vi "BPM-Chassis02 FPGA.vi"() -> ()   [LabVIEW 2011]
uses:
  <vilib>/rvi/eio/common/nirviEmuTemplateMethod_errors.vi
  <vilib>/rvi/Memory/Memory_Emulation/niFpgaMemoryEmulationValidateCache.vi
  <vilib>/rvi/DataTransferAndStorage/Container/Common/niFpgaContainerGetUniqueNameForEmu.vi
  <vilib>/rvi/Memory/Memory_Emulation/nirvimemoryEmulationManagerCache_InsertValue.vi
  <vilib>/Utility/error.llb/Clear Errors.vi
  <vilib>/rvi/Memory/Memory_Emulation/nirvimemoryEmulationManagerCache_GetValue.vi
  <vilib>/rvi/Memory/Memory_Emulation/nirvimemoryEmulationManagerCache_SetValue.vi
  <vilib>/eio/EIONode/EIONode.xnode
  <vilib>/eio/EIOMethodNode/EIOMethodNode.xnode
  <vilib>/rvi/DataTransferAndStorage/Container/XNode/niFpgaContainer.xnode
  <vilib>/rvi/Memory/Memory_Emulation/nirvimemoryEmulation.vi
panel:
  out "period":u32
  out "delay":u32
  out "dperiod":u32
  out "Timestamp":u32 caption="Tick Count(Ticks)"
  out "Mod3/AI3":fxp<+/-,20,5> format="%.17g"
  out "Mod3/AI2":fxp<+/-,20,5> format="%.17g"
  out "Mod1/AI1":fxp<+/-,20,5> format="%.17g"
  out "Mod2/AI3":fxp<+/-,20,5> format="%.17g"
  out "Mod2/AI2":fxp<+/-,20,5> format="%.17g"
  out "Mod2/AI1":fxp<+/-,20,5> format="%.17g"
  out "Mod2/AI0":fxp<+/-,20,5> format="%.17g"
  out "Mod1/AI3":fxp<+/-,20,5> format="%.17g"
  out "Mod1/AI2":fxp<+/-,20,5> format="%.17g"
  out "Mod1/AI0":fxp<+/-,20,5> format="%.17g"
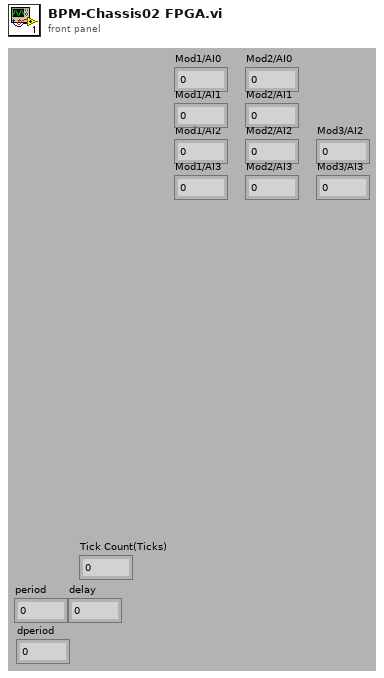
[diagram p1: front panel]
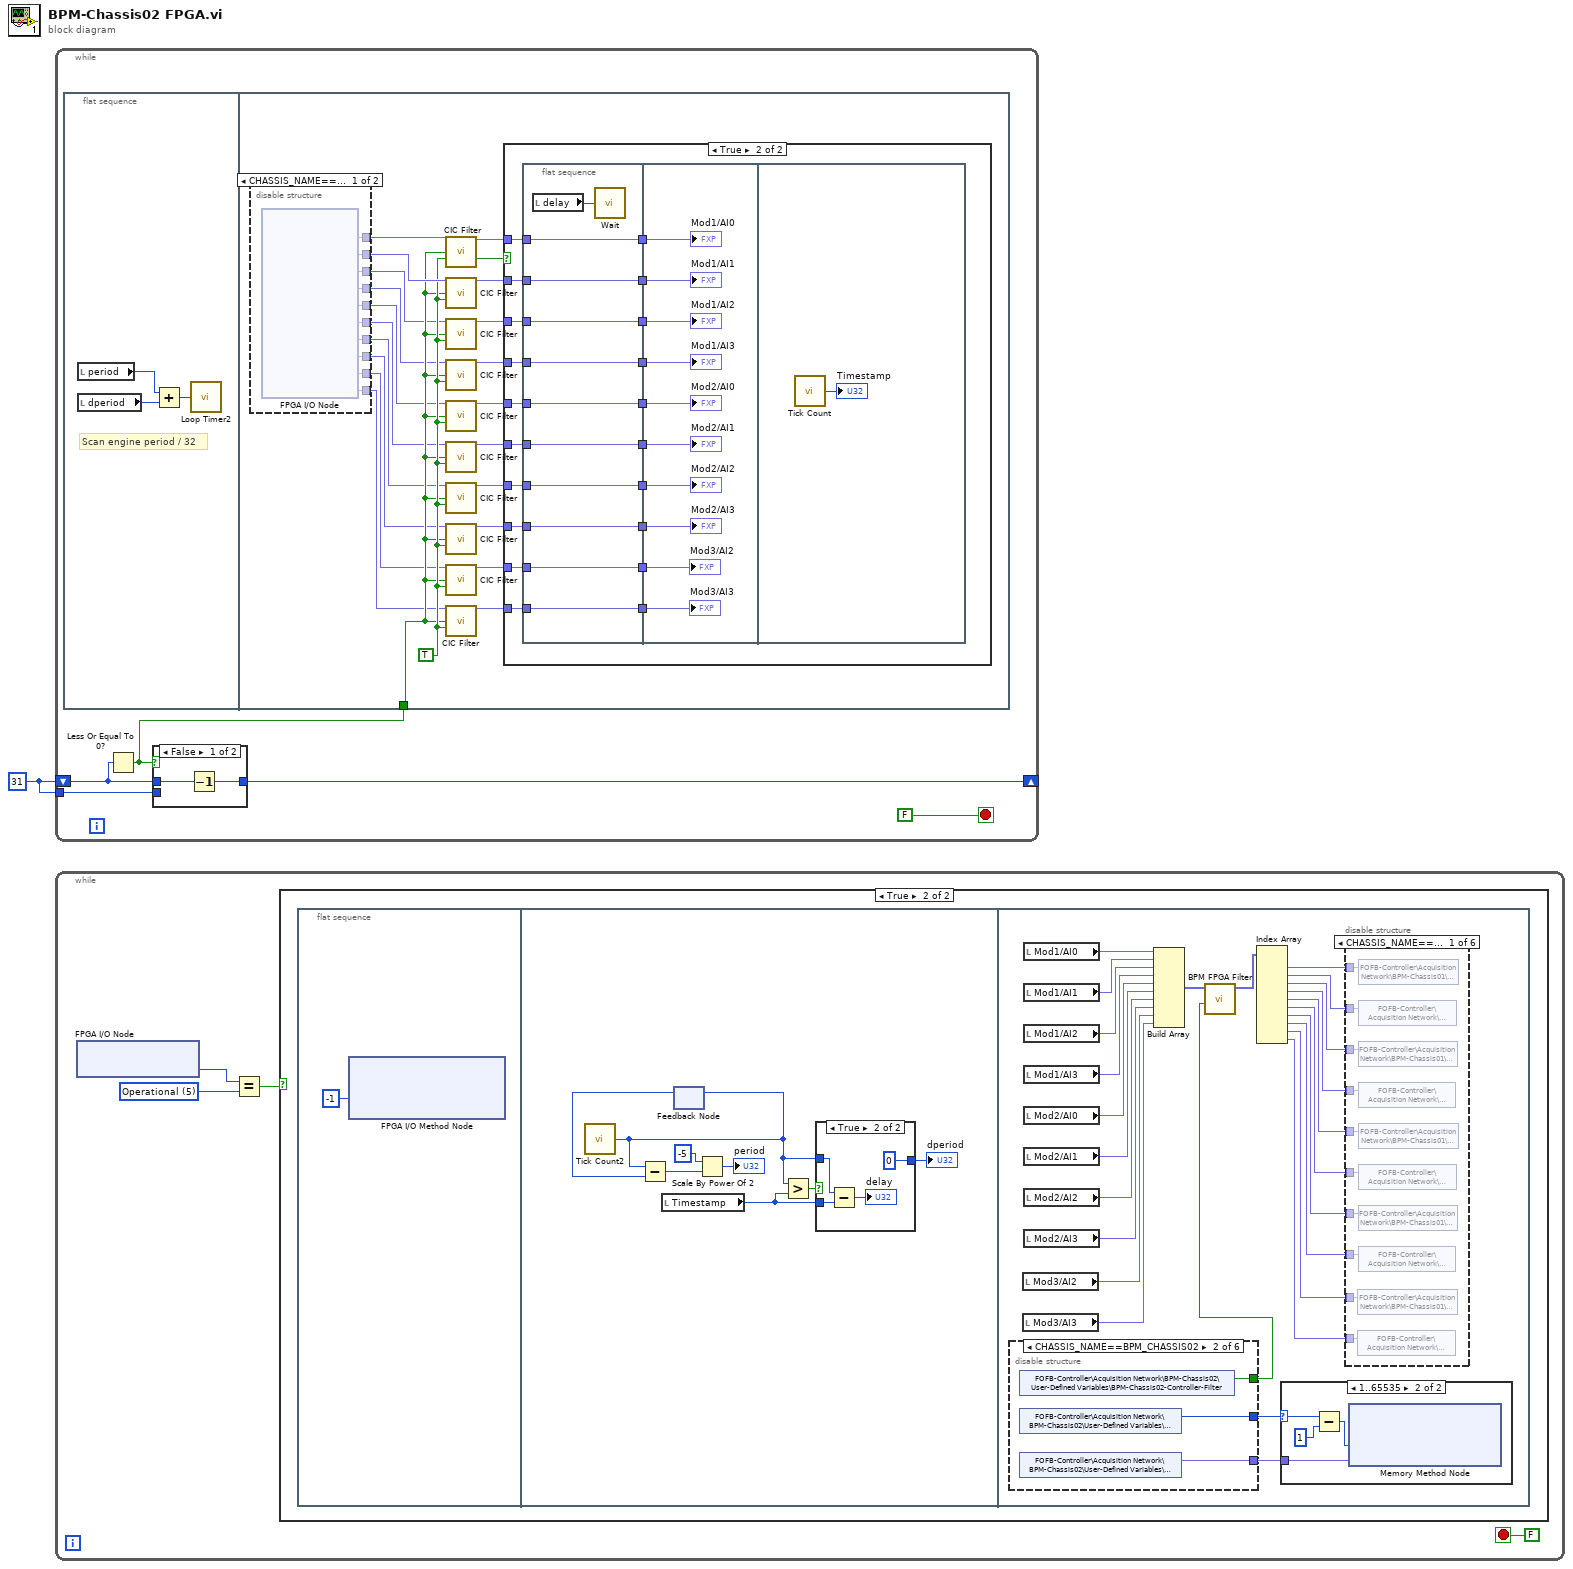
[diagram p0: block diagram]
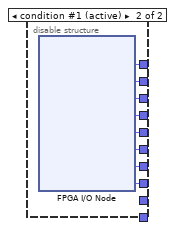
[diagram p3: hidden frame]
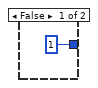
[diagram p6: hidden frame]
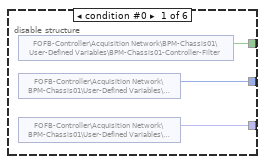
[diagram p8: hidden frame]
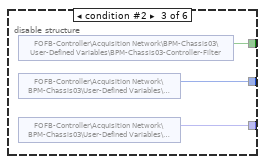
[diagram p9: hidden frame]
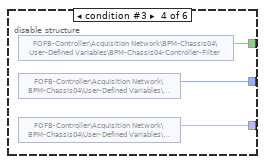
[diagram p10: hidden frame]
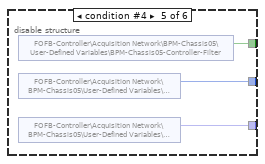
[diagram p11: hidden frame]
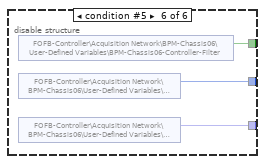
[diagram p12: hidden frame]
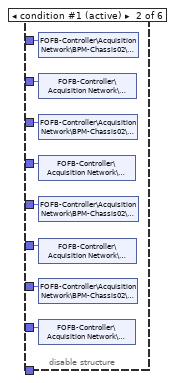
[diagram p13: hidden frame]
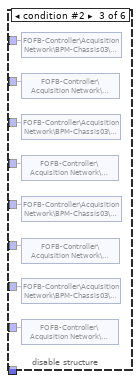
[diagram p14: hidden frame]
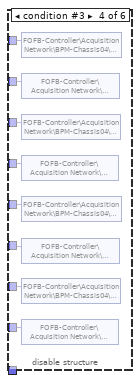
[diagram p15: hidden frame]
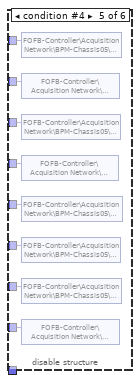
[diagram p16: hidden frame]
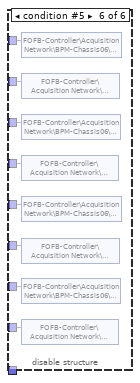
[diagram p17: hidden frame]
diagram:
  w1 = 31
  n1 = while {
    shift-right: [w5] -> _
    shift-left: w1 -> [w4]
    tunnel: w1 -> [w2]
    stop <- FALSE stop-if-true
    n2 = flat-sequence {
      tunnel: w3 -> [w30]
      frame #0 {
        # "Scan engine period / 32"
        n3 = local read "period"() -> (w12:u32)
        n4 = local read "dperiod"() -> (w11:u32)
        n5 = Add(x=w12, y=w11) -> (x+y=w10:u32)
        n6 = call "Loop Timer2"("Count(Ticks)"=w10) -> ()  [unwired: 1 out]
      }
      frame #1 {
        w31 = TRUE ("input valid")
        n7 = disable-structure shown="CHASSIS_NAME==BPM_CHASSIS01" {
          disable-tunnel: [w45 w53] -> w33
          disable-tunnel: [w44 w52] -> w32
          disable-tunnel: [w43 w51] -> w20
          disable-tunnel: [w42 w50] -> w19
          disable-tunnel: [w41 w49] -> w18
          disable-tunnel: [w40 w48] -> w17
          disable-tunnel: [w39 w47] -> w16
          disable-tunnel: [w38 w46] -> w15
          disable-tunnel: [w37 _] -> w14
          disable-tunnel: [w36 _] -> w13
          frame condition #0 {
            n8 = xnode "FPGA I/O Node"() -> ("Mod1/AI0"=w45:fxp<+/-,20,5>, "Mod1/AI1"=w44:fxp<+/-,20,5>, "Mod1/AI2"=w43:fxp<+/-,20,5>, "Mod1/AI3"=w42:fxp<+/-,20,5>, "Mod2/AI0"=w41:fxp<+/-,20,5>, "Mod2/AI1"=w40:fxp<+/-,20,5>, "Mod2/AI2"=w39:fxp<+/-,20,5>, "Mod2/AI3"=w38:fxp<+/-,20,5>, "Mod3/AI2"=w37, "Mod3/AI3"=w36)  [unwired: 10 in, 10 out]
          }
          frame condition #1 (active) {
            n9 = xnode "FPGA I/O Node"() -> ("Mod1/AI0"=w53:fxp<+/-,20,5>, "Mod1/AI1"=w52:fxp<+/-,20,5>, "Mod1/AI2"=w51:fxp<+/-,20,5>, "Mod1/AI3"=w50:fxp<+/-,20,5>, "Mod2/AI0"=w49:fxp<+/-,20,5>, "Mod2/AI1"=w48:fxp<+/-,20,5>, "Mod2/AI2"=w47:fxp<+/-,20,5>, "Mod2/AI3"=w46:fxp<+/-,20,5>)  [unwired: 8 in, 8 out]
          }
        }
        n10 = call "CIC Filter.vi"("input data"=w33, "sample"=w30, "input valid"=w31) -> ("output data"=w34:fxp<+/-,20,5>, "output valid"=w35:bool)  [unwired: 10 in, 1 out]
        n11 = call "CIC Filter.vi"("input data"=w32, "sample"=w30, "input valid"=w31) -> ("output data"=w29:fxp<+/-,20,5>)  [unwired: 10 in, 2 out]
        n12 = call "CIC Filter.vi"("input data"=w20, "sample"=w30, "input valid"=w31) -> ("output data"=w28:fxp<+/-,20,5>)  [unwired: 10 in, 2 out]
        n13 = call "CIC Filter.vi"("input data"=w19, "sample"=w30, "input valid"=w31) -> ("output data"=w27:fxp<+/-,20,5>)  [unwired: 10 in, 2 out]
        n14 = call "CIC Filter.vi"("input data"=w18, "sample"=w30, "input valid"=w31) -> ("output data"=w26:fxp<+/-,20,5>)  [unwired: 10 in, 2 out]
        n15 = call "CIC Filter.vi"("input data"=w17, "sample"=w30, "input valid"=w31) -> ("output data"=w25:fxp<+/-,20,5>)  [unwired: 10 in, 2 out]
        n16 = call "CIC Filter.vi"("input data"=w16, "sample"=w30, "input valid"=w31) -> ("output data"=w24:fxp<+/-,20,5>)  [unwired: 10 in, 2 out]
        n17 = call "CIC Filter.vi"("input data"=w15, "sample"=w30, "input valid"=w31) -> ("output data"=w23:fxp<+/-,20,5>)  [unwired: 10 in, 2 out]
        n18 = call "CIC Filter.vi"("input data"=w14, "sample"=w30, "input valid"=w31) -> ("output data"=w22:fxp<+/-,20,5>)  [unwired: 10 in, 2 out]
        n19 = call "CIC Filter.vi"("input data"=w13, "sample"=w30, "input valid"=w31) -> ("output data"=w21:fxp<+/-,20,5>)  [unwired: 10 in, 2 out]
        n20 = case shown="True" w35 {
          tunnel: w34 -> [_ w73]
          tunnel: w29 -> [_ w71]
          tunnel: w28 -> [_ w69]
          tunnel: w27 -> [_ w68]
          tunnel: w26 -> [_ w65]
          tunnel: w25 -> [_ w63]
          tunnel: w24 -> [_ w61]
          tunnel: w23 -> [_ w59]
          tunnel: w22 -> [_ w57]
          tunnel: w21 -> [_ w55]
          frame False {
          }
          frame True {
            n21 = flat-sequence {
              tunnel: w73 -> [w84]
              tunnel: [w84] -> w72
              tunnel: w71 -> [w82]
              tunnel: [w82] -> w70
              tunnel: w69 -> [w80]
              tunnel: w68 -> [w81]
              tunnel: [w81] -> w67
              tunnel: [w80] -> w66
              tunnel: w65 -> [w79]
              tunnel: [w79] -> w64
              tunnel: w63 -> [w78]
              tunnel: [w78] -> w62
              tunnel: w61 -> [w77]
              tunnel: [w77] -> w60
              tunnel: w59 -> [w76]
              tunnel: [w76] -> w58
              tunnel: w57 -> [w75]
              tunnel: [w75] -> w56
              tunnel: w55 -> [w74]
              tunnel: [w74] -> w54
              tunnel: w72 -> [w93]
              tunnel: w70 -> [w94]
              tunnel: w67 -> [w92]
              tunnel: w66 -> [w91]
              tunnel: w64 -> [w90]
              tunnel: w62 -> [w89]
              tunnel: w60 -> [w88]
              tunnel: w58 -> [w87]
              tunnel: w56 -> [w86]
              tunnel: w54 -> [w85]
              frame #0 {
                n22 = local read "delay"() -> (w83:u32)
                n23 = call "Wait"("Count(Ticks)"=w83) -> ()  [unwired: 1 out]
              }
              frame #1 {
                "Mod1/AI0" <- w93
                "Mod1/AI2" <- w91
                "Mod1/AI3" <- w92
                "Mod2/AI0" <- w90
                "Mod2/AI1" <- w89
                "Mod2/AI2" <- w88
                "Mod2/AI3" <- w87
                "Mod1/AI1" <- w94
                "Mod3/AI2" <- w86
                "Mod3/AI3" <- w85
              }
              frame #2 {
                n24 = call "Tick Count"() -> ("Tick Count(Ticks)"=→"Timestamp":u32)
              }
            }
          }
        }
      }
    }
    n25 = Less Or Equal To 0?(x=w4) -> (x <= 0?=w3:bool)
    n26 = case shown="False" w3 {
      tunnel: [w8 w9] -> w5
      tunnel: w4 -> [w7 _]
      tunnel: w2 -> [_ w9]
      frame False {
        n27 = Decrement(x=w7) -> (x-1=w8:i32)
      }
      frame True {
      }
    }
  }
  n28 = while {
    stop <- FALSE stop-if-true
    w98 = u8 5 items=["Init"=1, "PreOp"=2, "Bootstrap"=3, "SafeOp"=4, "Operational"=5]
    n29 = xnode "FPGA I/O Node"() -> ("EtherCAT State"=w97:u8)  [unwired: 1 in, 1 out]
    n30 = Equal?(x=w97, y=w98) -> (x = y?=w96:bool)
    n31 = case shown="True" w96 {
      frame False {
      }
      frame True {
        n32 = flat-sequence {
          frame #0 {
            n33 = xnode "FPGA I/O Method Node"("Timeout"=-1) -> ()  [unwired: 1 in, 2 out]
          }
          frame #1 {
            n34 = call "Tick Count2"() -> ("Tick Count(Ticks)"=w102:u32)
            n35 = local read "Timestamp"() -> (w104:u32)
            n36 = feedback #1() -> (w101:u32)  [unwired: 1 in]
            n37 = Subtract(x=w102, y=w101) -> (x-y=w107:u32)
            n38 = feedback-in #1(w102) -> ()
            n39 = Scale By Power Of 2(n=i8 -5, x=w107) -> (x*2^n=→"period":u32)
            n40 = Greater?(x=w102, y=w104) -> (0:w105:bool)
            n41 = case shown="True" w105 {
              tunnel: w102 -> [_ w113]
              tunnel: w104 -> [_ w112]
              tunnel: [u32 1 ("dt 2") u32 0 ("dt 2")] -> w103
              frame False {
              }
              frame True {
                n42 = Subtract(x=w113, y=w112) -> (x-y=→"delay":u32)
              }
            }
            "dperiod" <- w103
          }
          frame #2 {
            n43 = disable-structure shown="CHASSIS_NAME==BPM_CHASSIS02" {
              disable-tunnel: [w145 w147 w150 w153 w155 w159] -> w115
              disable-tunnel: [w144 w146 w149 w152 w156 w158] -> w114
              disable-tunnel: [w143 w148 w151 w154 w157 w160] -> w116
              frame condition #0 {
                n44 = shared-variable "FOFB-Controller\\Acquisition Network\\BPM-Chassis01\\User-Defined Variables\\BPM-Chassis01-Controller-Filter"() -> (w143:bool)  [unwired: 1 in, 1 out]
                n45 = shared-variable "FOFB-Controller\\Acquisition Network\\BPM-Chassis01\\User-Defined Variables\\BPM-Chassis01-ADDR"() -> (w145:u16)  [unwired: 1 in, 1 out]
                n46 = shared-variable "FOFB-Controller\\Acquisition Network\\BPM-Chassis01\\User-Defined Variables\\BPM-Chassis01-DATA"() -> (w144:fxp<+/-,22,4>)  [unwired: 1 in, 1 out]
              }
              frame condition #1 (active) {
                n47 = shared-variable "FOFB-Controller\\Acquisition Network\\BPM-Chassis02\\User-Defined Variables\\BPM-Chassis02-Controller-Filter"() -> (w148:bool)  [unwired: 1 in, 1 out]
                n48 = shared-variable "FOFB-Controller\\Acquisition Network\\BPM-Chassis02\\User-Defined Variables\\BPM-Chassis02-ADDR"() -> (w147:u16)  [unwired: 1 in, 1 out]
                n49 = shared-variable "FOFB-Controller\\Acquisition Network\\BPM-Chassis02\\User-Defined Variables\\BPM-Chassis02-DATA"() -> (w146:fxp<+/-,22,4>)  [unwired: 1 in, 1 out]
              }
              frame condition #2 {
                n50 = shared-variable "FOFB-Controller\\Acquisition Network\\BPM-Chassis03\\User-Defined Variables\\BPM-Chassis03-Controller-Filter"() -> (w151:bool)  [unwired: 1 in, 1 out]
                n51 = shared-variable "FOFB-Controller\\Acquisition Network\\BPM-Chassis03\\User-Defined Variables\\BPM-Chassis03-ADDR"() -> (w150:u16)  [unwired: 1 in, 1 out]
                n52 = shared-variable "FOFB-Controller\\Acquisition Network\\BPM-Chassis03\\User-Defined Variables\\BPM-Chassis03-DATA"() -> (w149:fxp<+/-,22,4>)  [unwired: 1 in, 1 out]
              }
              frame condition #3 {
                n53 = shared-variable "FOFB-Controller\\Acquisition Network\\BPM-Chassis04\\User-Defined Variables\\BPM-Chassis04-Controller-Filter"() -> (w154:bool)  [unwired: 1 in, 1 out]
                n54 = shared-variable "FOFB-Controller\\Acquisition Network\\BPM-Chassis04\\User-Defined Variables\\BPM-Chassis04-ADDR"() -> (w153:u16)  [unwired: 1 in, 1 out]
                n55 = shared-variable "FOFB-Controller\\Acquisition Network\\BPM-Chassis04\\User-Defined Variables\\BPM-Chassis04-DATA"() -> (w152:fxp<+/-,22,4>)  [unwired: 1 in, 1 out]
              }
              frame condition #4 {
                n56 = shared-variable "FOFB-Controller\\Acquisition Network\\BPM-Chassis05\\User-Defined Variables\\BPM-Chassis05-Controller-Filter"() -> (w157:bool)  [unwired: 1 in, 1 out]
                n57 = shared-variable "FOFB-Controller\\Acquisition Network\\BPM-Chassis05\\User-Defined Variables\\BPM-Chassis05-ADDR"() -> (w155:u16)  [unwired: 1 in, 1 out]
                n58 = shared-variable "FOFB-Controller\\Acquisition Network\\BPM-Chassis05\\User-Defined Variables\\BPM-Chassis05-DATA"() -> (w156:fxp<+/-,22,4>)  [unwired: 1 in, 1 out]
              }
              frame condition #5 {
                n59 = shared-variable "FOFB-Controller\\Acquisition Network\\BPM-Chassis06\\User-Defined Variables\\BPM-Chassis06-Controller-Filter"() -> (w160:bool)  [unwired: 1 in, 1 out]
                n60 = shared-variable "FOFB-Controller\\Acquisition Network\\BPM-Chassis06\\User-Defined Variables\\BPM-Chassis06-ADDR"() -> (w159:u16)  [unwired: 1 in, 1 out]
                n61 = shared-variable "FOFB-Controller\\Acquisition Network\\BPM-Chassis06\\User-Defined Variables\\BPM-Chassis06-DATA"() -> (w158:fxp<+/-,22,4>)  [unwired: 1 in, 1 out]
              }
            }
            n62 = local read "Mod3/AI2"() -> (w120:fxp<+/-,20,5>)
            n63 = local read "Mod3/AI3"() -> (w119:fxp<+/-,20,5>)
            n64 = local read "Mod1/AI0"() -> (w138:fxp<+/-,20,5>)
            n65 = local read "Mod1/AI1"() -> (w137:fxp<+/-,20,5>)
            n66 = local read "Mod1/AI2"() -> (w136:fxp<+/-,20,5>)
            n67 = local read "Mod1/AI3"() -> (w135:fxp<+/-,20,5>)
            n68 = local read "Mod2/AI0"() -> (w134:fxp<+/-,20,5>)
            n69 = local read "Mod2/AI1"() -> (w133:fxp<+/-,20,5>)
            n70 = local read "Mod2/AI2"() -> (w132:fxp<+/-,20,5>)
            n71 = local read "Mod2/AI3"() -> (w131:fxp<+/-,20,5>)
            n72 = Build Array(w138, w137, w136, w135, w134, w133, w132, w131, w120, w119) -> (w130:fxp<+/-,20,5>[])
            n73 = call "BPM FPGA Filter.vi"("filter?"=w116, "input"=w130) -> ("output"=w129:fxp<+/-,20,5>[])  [unwired: 8 in, 1 out]
            n74 = Index Array(array=w129) -> (element #1=w128:fxp<+/-,20,5>, element #2=w127:fxp<+/-,20,5>, element #3=w126:fxp<+/-,20,5>, element #4=w125:fxp<+/-,20,5>, element #5=w124:fxp<+/-,20,5>, element #6=w123:fxp<+/-,20,5>, element #7=w122:fxp<+/-,20,5>, element #8=w121:fxp<+/-,20,5>, element #9=w118:fxp<+/-,20,5>, element #10=w117:fxp<+/-,20,5>)  [unwired: 10 in]
            n75 = case shown="1..65535" w115 {
              selector: w115 -> [_ w142]
              tunnel: w114 -> [_ w139]
              frame 0, Default {
              }
              frame 1..65535 {
                n76 = Subtract(x=w142, y=u16 1) -> (x-y=w140:u16)
                n77 = xnode ("Memory Method Node")("Address"=w140, "Data"=w139) -> ()  [unwired: 1 in, 1 out]
              }
            }
            n78 = disable-structure shown="CHASSIS_NAME==BPM_CHASSIS01, default" {
              disable-tunnel: w118 -> [w170 _ _ _ _ _]
              disable-tunnel: w117 -> [w169 _ _ _ _ _]
              disable-tunnel: w128 -> [w168 w178 w186 w194 w202 w210]
              disable-tunnel: w127 -> [w167 w177 w185 w193 w201 w209]
              disable-tunnel: w126 -> [w166 w176 w184 w192 w200 w208]
              disable-tunnel: w125 -> [w165 w175 w183 w191 w199 w207]
              disable-tunnel: w124 -> [w164 w174 w182 w190 w198 w206]
              disable-tunnel: w123 -> [w163 w173 w181 w189 w197 w205]
              disable-tunnel: w122 -> [w162 w172 w180 w188 w196 w204]
              disable-tunnel: w121 -> [w161 w171 w179 w187 w195 w203]
              frame condition #0 {
                n79 = shared-variable "FOFB-Controller\\Acquisition Network\\BPM-Chassis01\\User-Defined Variables\\AMP03CH"(w170) -> ()  [unwired: 1 in, 1 out]
                n80 = shared-variable "FOFB-Controller\\Acquisition Network\\BPM-Chassis01\\User-Defined Variables\\AMP03CV"(w169) -> ()  [unwired: 1 in, 1 out]
                n81 = shared-variable "FOFB-Controller\\Acquisition Network\\BPM-Chassis01\\User-Defined Variables\\AMP02AH"(w168) -> ()  [unwired: 1 in, 1 out]
                n82 = shared-variable "FOFB-Controller\\Acquisition Network\\BPM-Chassis01\\User-Defined Variables\\AMP02AV"(w167) -> ()  [unwired: 1 in, 1 out]
                n83 = shared-variable "FOFB-Controller\\Acquisition Network\\BPM-Chassis01\\User-Defined Variables\\AMP02BH"(w166) -> ()  [unwired: 1 in, 1 out]
                n84 = shared-variable "FOFB-Controller\\Acquisition Network\\BPM-Chassis01\\User-Defined Variables\\AMP02BV"(w165) -> ()  [unwired: 1 in, 1 out]
                n85 = shared-variable "FOFB-Controller\\Acquisition Network\\BPM-Chassis01\\User-Defined Variables\\AMP03AH"(w164) -> ()  [unwired: 1 in, 1 out]
                n86 = shared-variable "FOFB-Controller\\Acquisition Network\\BPM-Chassis01\\User-Defined Variables\\AMP03AV"(w163) -> ()  [unwired: 1 in, 1 out]
                n87 = shared-variable "FOFB-Controller\\Acquisition Network\\BPM-Chassis01\\User-Defined Variables\\AMP03BH"(w162) -> ()  [unwired: 1 in, 1 out]
                n88 = shared-variable "FOFB-Controller\\Acquisition Network\\BPM-Chassis01\\User-Defined Variables\\AMP03BV"(w161) -> ()  [unwired: 1 in, 1 out]
              }
              frame condition #1 (active) {
                n89 = shared-variable "FOFB-Controller\\Acquisition Network\\BPM-Chassis02\\User-Defined Variables\\AMP04AH"(w178) -> ()  [unwired: 1 in, 1 out]
                n90 = shared-variable "FOFB-Controller\\Acquisition Network\\BPM-Chassis02\\User-Defined Variables\\AMP04AV"(w177) -> ()  [unwired: 1 in, 1 out]
                n91 = shared-variable "FOFB-Controller\\Acquisition Network\\BPM-Chassis02\\User-Defined Variables\\AMP04BH"(w176) -> ()  [unwired: 1 in, 1 out]
                n92 = shared-variable "FOFB-Controller\\Acquisition Network\\BPM-Chassis02\\User-Defined Variables\\AMP04BV"(w175) -> ()  [unwired: 1 in, 1 out]
                n93 = shared-variable "FOFB-Controller\\Acquisition Network\\BPM-Chassis02\\User-Defined Variables\\AMP05AH"(w174) -> ()  [unwired: 1 in, 1 out]
                n94 = shared-variable "FOFB-Controller\\Acquisition Network\\BPM-Chassis02\\User-Defined Variables\\AMP05AV"(w173) -> ()  [unwired: 1 in, 1 out]
                n95 = shared-variable "FOFB-Controller\\Acquisition Network\\BPM-Chassis02\\User-Defined Variables\\AMP05BH"(w172) -> ()  [unwired: 1 in, 1 out]
                n96 = shared-variable "FOFB-Controller\\Acquisition Network\\BPM-Chassis02\\User-Defined Variables\\AMP05BV"(w171) -> ()  [unwired: 1 in, 1 out]
              }
              frame condition #2 {
                n97 = shared-variable "FOFB-Controller\\Acquisition Network\\BPM-Chassis03\\User-Defined Variables\\AMP06AH"(w186) -> ()  [unwired: 1 in, 1 out]
                n98 = shared-variable "FOFB-Controller\\Acquisition Network\\BPM-Chassis03\\User-Defined Variables\\AMP06AV"(w185) -> ()  [unwired: 1 in, 1 out]
                n99 = shared-variable "FOFB-Controller\\Acquisition Network\\BPM-Chassis03\\User-Defined Variables\\AMP06BH"(w184) -> ()  [unwired: 1 in, 1 out]
                n100 = shared-variable "FOFB-Controller\\Acquisition Network\\BPM-Chassis03\\User-Defined Variables\\AMP06BV"(w183) -> ()  [unwired: 1 in, 1 out]
                n101 = shared-variable "FOFB-Controller\\Acquisition Network\\BPM-Chassis03\\User-Defined Variables\\AMP07AH"(w182) -> ()  [unwired: 1 in, 1 out]
                n102 = shared-variable "FOFB-Controller\\Acquisition Network\\BPM-Chassis03\\User-Defined Variables\\AMP07AV"(w181) -> ()  [unwired: 1 in, 1 out]
                n103 = shared-variable "FOFB-Controller\\Acquisition Network\\BPM-Chassis03\\User-Defined Variables\\AMP07BH"(w180) -> ()  [unwired: 1 in, 1 out]
                n104 = shared-variable "FOFB-Controller\\Acquisition Network\\BPM-Chassis03\\User-Defined Variables\\AMP07BV"(w179) -> ()  [unwired: 1 in, 1 out]
              }
              frame condition #3 {
                n105 = shared-variable "FOFB-Controller\\Acquisition Network\\BPM-Chassis04\\User-Defined Variables\\AMP08AH"(w194) -> ()  [unwired: 1 in, 1 out]
                n106 = shared-variable "FOFB-Controller\\Acquisition Network\\BPM-Chassis04\\User-Defined Variables\\AMP08AV"(w193) -> ()  [unwired: 1 in, 1 out]
                n107 = shared-variable "FOFB-Controller\\Acquisition Network\\BPM-Chassis04\\User-Defined Variables\\AMP08BH"(w192) -> ()  [unwired: 1 in, 1 out]
                n108 = shared-variable "FOFB-Controller\\Acquisition Network\\BPM-Chassis04\\User-Defined Variables\\AMP08BV"(w191) -> ()  [unwired: 1 in, 1 out]
                n109 = shared-variable "FOFB-Controller\\Acquisition Network\\BPM-Chassis04\\User-Defined Variables\\AMP09AH"(w190) -> ()  [unwired: 1 in, 1 out]
                n110 = shared-variable "FOFB-Controller\\Acquisition Network\\BPM-Chassis04\\User-Defined Variables\\AMP09AV"(w189) -> ()  [unwired: 1 in, 1 out]
                n111 = shared-variable "FOFB-Controller\\Acquisition Network\\BPM-Chassis04\\User-Defined Variables\\AMP09BH"(w188) -> ()  [unwired: 1 in, 1 out]
                n112 = shared-variable "FOFB-Controller\\Acquisition Network\\BPM-Chassis04\\User-Defined Variables\\AMP09BV"(w187) -> ()  [unwired: 1 in, 1 out]
              }
              frame condition #4 {
                n113 = shared-variable "FOFB-Controller\\Acquisition Network\\BPM-Chassis05\\User-Defined Variables\\AMP10AH"(w202) -> ()  [unwired: 1 in, 1 out]
                n114 = shared-variable "FOFB-Controller\\Acquisition Network\\BPM-Chassis05\\User-Defined Variables\\AMP10AV"(w201) -> ()  [unwired: 1 in, 1 out]
                n115 = shared-variable "FOFB-Controller\\Acquisition Network\\BPM-Chassis05\\User-Defined Variables\\AMP10BH"(w200) -> ()  [unwired: 1 in, 1 out]
                n116 = shared-variable "FOFB-Controller\\Acquisition Network\\BPM-Chassis05\\User-Defined Variables\\AMP10BV"(w199) -> ()  [unwired: 1 in, 1 out]
                n117 = shared-variable "FOFB-Controller\\Acquisition Network\\BPM-Chassis05\\User-Defined Variables\\AMU11AH"(w198) -> ()  [unwired: 1 in, 1 out]
                n118 = shared-variable "FOFB-Controller\\Acquisition Network\\BPM-Chassis05\\User-Defined Variables\\AMU11AV"(w197) -> ()  [unwired: 1 in, 1 out]
                n119 = shared-variable "FOFB-Controller\\Acquisition Network\\BPM-Chassis05\\User-Defined Variables\\AMU11BH"(w196) -> ()  [unwired: 1 in, 1 out]
                n120 = shared-variable "FOFB-Controller\\Acquisition Network\\BPM-Chassis05\\User-Defined Variables\\AMU11BV"(w195) -> ()  [unwired: 1 in, 1 out]
              }
              frame condition #5 {
                n121 = shared-variable "FOFB-Controller\\Acquisition Network\\BPM-Chassis06\\User-Defined Variables\\AMP12AH"(w210) -> ()  [unwired: 1 in, 1 out]
                n122 = shared-variable "FOFB-Controller\\Acquisition Network\\BPM-Chassis06\\User-Defined Variables\\AMP12AV"(w209) -> ()  [unwired: 1 in, 1 out]
                n123 = shared-variable "FOFB-Controller\\Acquisition Network\\BPM-Chassis06\\User-Defined Variables\\AMP12BH"(w208) -> ()  [unwired: 1 in, 1 out]
                n124 = shared-variable "FOFB-Controller\\Acquisition Network\\BPM-Chassis06\\User-Defined Variables\\AMP12BV"(w207) -> ()  [unwired: 1 in, 1 out]
                n125 = shared-variable "FOFB-Controller\\Acquisition Network\\BPM-Chassis06\\User-Defined Variables\\AMP01AH"(w206) -> ()  [unwired: 1 in, 1 out]
                n126 = shared-variable "FOFB-Controller\\Acquisition Network\\BPM-Chassis06\\User-Defined Variables\\AMP01AV"(w205) -> ()  [unwired: 1 in, 1 out]
                n127 = shared-variable "FOFB-Controller\\Acquisition Network\\BPM-Chassis06\\User-Defined Variables\\AMP01BH"(w204) -> ()  [unwired: 1 in, 1 out]
                n128 = shared-variable "FOFB-Controller\\Acquisition Network\\BPM-Chassis06\\User-Defined Variables\\AMP01BV"(w203) -> ()  [unwired: 1 in, 1 out]
              }
            }
          }
        }
      }
    }
  }
